vi "Reset-log.vi"(8 "error in (no error)":errorcluster, 11 "Errors in":T1) -> (0 "error out":errorcluster, 3 "Errors out":T1)   [LabVIEW 2013, in "Error-handling.lvlib" / "Errors.lvclass"]
uses:
  Errors.lvclass
  Object-reference.ctl
  Errors.lvclass/Errors.ctl
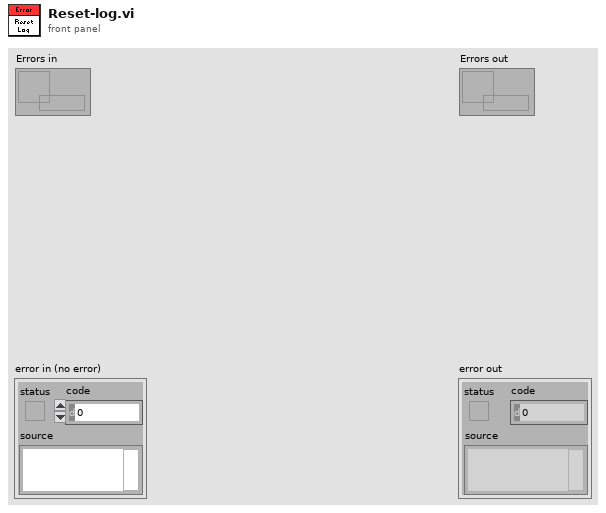
[diagram p1: front panel]
types:
  T1 = typedef "Error-handling.lvlib/Errors.lvclass/Object-reference.ctl" = refnum<data-value>
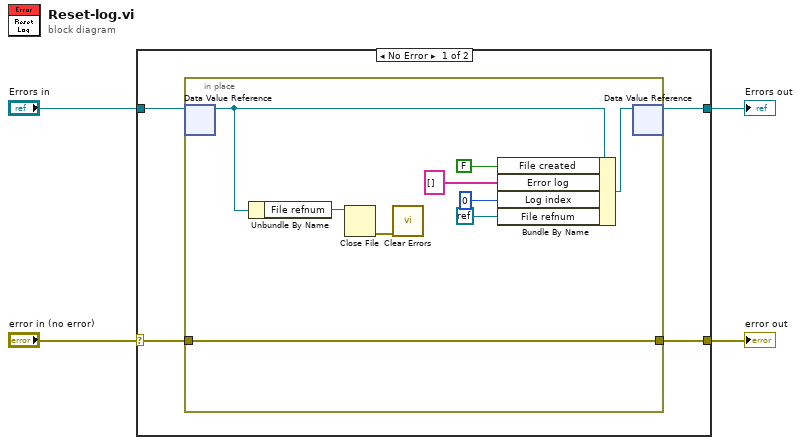
[diagram p0: block diagram]
diagram:
  n1 = case shown="No Error" "error in (no error)" {
    selector: "error in (no error)" -> [w8 w19]
    tunnel: [w7 w19] -> w3
    tunnel: [w5 w18] -> w1
    tunnel: "Errors in" -> [w6 w18]
    frame No Error {
      n2 = in-place {
        in-place-border: w8 -> [w12]
        in-place-border: [w12] -> w7
        n3 = in-place-dvr #1(w6) -> (w11:refnum<class "Errors.lvclass">)  [unwired: 1 out]
        n4 = Unbundle By Name(w11) -> ("File refnum"=w10:refnum<file>)
        n5 = Close File(refnum=w10) -> (error out=w9:errorcluster)  [unwired: 1 in, 1 out]
        n6 = call <vilib>:"Clear Errors.vi"("error in (no error)"=w9) -> ()  [unwired: 6 in, 1 out]
        n7 = Bundle By Name(cluster=w11, "File created"=FALSE ("Status.File created"), "Error log"=string[] [], "Log index"=0, "File refnum"=refnum<k0> refnum) -> (w17:refnum<class "Errors.lvclass">)
        n8 = in-place-dvr #1(w17) -> (w5:T1)  [unwired: 1 out]
      }
    }
    frame Error {
    }
  }
  "error out" <- w3
  "Errors out" <- w1
